vi "BlobSearch.vi"(1 "BlobData R":T2(array[cluster]), 2 "BlobData L":T2(array[cluster])) -> (0 "BlobData":T1(array[cluster]))   [LabVIEW 2011]
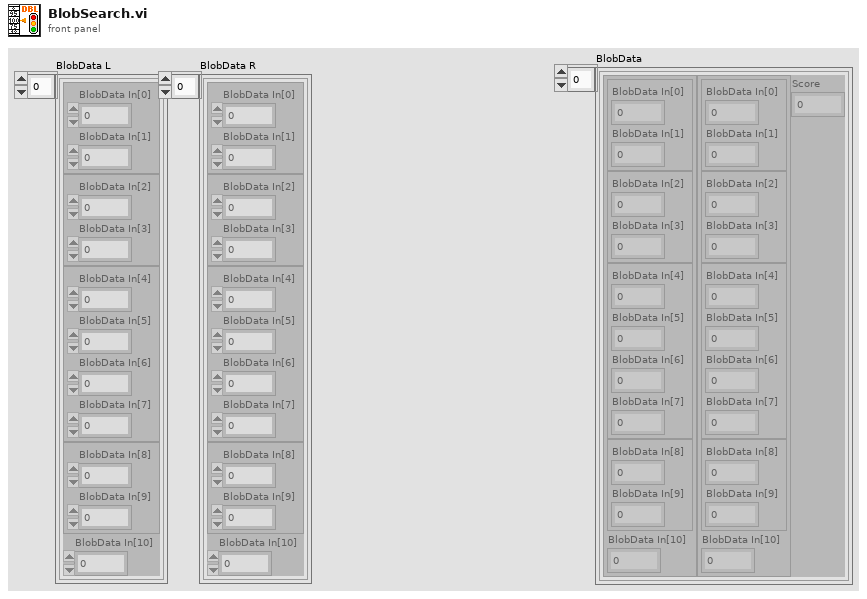
[diagram p1: front panel]
types:
  T1 = cluster{cluster{cluster{"BlobData In[0]":dbl, "BlobData In[1]":dbl}, cluster{"BlobData In[2]":dbl, "BlobData In[3]":dbl}, cluster{"BlobData In[4]":dbl, "BlobData In[5]":dbl, "BlobData In[6]":dbl, "BlobData In[7]":dbl}, cluster{"BlobData In[8]":dbl, "BlobData In[9]":dbl}, "BlobData In[10]":dbl}, cluster{cluster{"BlobData In[0]":dbl, "BlobData In[1]":dbl}, cluster{"BlobData In[2]":dbl, "BlobData In[3]":dbl}, cluster{"BlobData In[4]":dbl, "BlobData In[5]":dbl, "BlobData In[6]":dbl, "BlobData In[7]":dbl}, cluster{"BlobData In[8]":dbl, "BlobData In[9]":dbl}, "BlobData In[10]":dbl}, "Score":dbl}[]
  T2 = cluster{cluster{"BlobData In[0]":dbl, "BlobData In[1]":dbl}, cluster{"BlobData In[2]":dbl, "BlobData In[3]":dbl}, cluster{"BlobData In[4]":dbl, "BlobData In[5]":dbl, "BlobData In[6]":dbl, "BlobData In[7]":dbl}, cluster{"BlobData In[8]":dbl, "BlobData In[9]":dbl}, "BlobData In[10]":dbl}[]
  T3 = cluster{cluster{cluster{"BlobData In[0]":dbl, "BlobData In[1]":dbl}, cluster{"BlobData In[2]":dbl, "BlobData In[3]":dbl}, cluster{"BlobData In[4]":dbl, "BlobData In[5]":dbl, "BlobData In[6]":dbl, "BlobData In[7]":dbl}, cluster{"BlobData In[8]":dbl, "BlobData In[9]":dbl}, "BlobData In[10]":dbl}, cluster{cluster{"BlobData In[0]":dbl, "BlobData In[1]":dbl}, cluster{"BlobData In[2]":dbl, "BlobData In[3]":dbl}, cluster{"BlobData In[4]":dbl, "BlobData In[5]":dbl, "BlobData In[6]":dbl, "BlobData In[7]":dbl}, cluster{"BlobData In[8]":dbl, "BlobData In[9]":dbl}, "BlobData In[10]":dbl}, dbl}[]
  T4 = cluster{cluster{"BlobData In[0]":dbl, "BlobData In[1]":dbl}, cluster{"BlobData In[2]":dbl, "BlobData In[3]":dbl}, cluster{"BlobData In[4]":dbl, "BlobData In[5]":dbl, "BlobData In[6]":dbl, "BlobData In[7]":dbl}, cluster{"BlobData In[8]":dbl, "BlobData In[9]":dbl}, "BlobData In[10]":dbl}
  T5 = cluster{"BlobData In[0]":dbl, "BlobData In[1]":dbl}
  T6 = cluster{"BlobData In[2]":dbl, "BlobData In[3]":dbl}
  T7 = cluster{"BlobData In[4]":dbl, "BlobData In[5]":dbl, "BlobData In[6]":dbl, "BlobData In[7]":dbl}
  T8 = cluster{"BlobData In[8]":dbl, "BlobData In[9]":dbl}
  T9 = cluster{cluster{cluster{"BlobData In[0]":dbl, "BlobData In[1]":dbl}, cluster{"BlobData In[2]":dbl, "BlobData In[3]":dbl}, cluster{"BlobData In[4]":dbl, "BlobData In[5]":dbl, "BlobData In[6]":dbl, "BlobData In[7]":dbl}, cluster{"BlobData In[8]":dbl, "BlobData In[9]":dbl}, "BlobData In[10]":dbl}, cluster{cluster{"BlobData In[0]":dbl, "BlobData In[1]":dbl}, cluster{"BlobData In[2]":dbl, "BlobData In[3]":dbl}, cluster{"BlobData In[4]":dbl, "BlobData In[5]":dbl, "BlobData In[6]":dbl, "BlobData In[7]":dbl}, cluster{"BlobData In[8]":dbl, "BlobData In[9]":dbl}, "BlobData In[10]":dbl}, dbl}
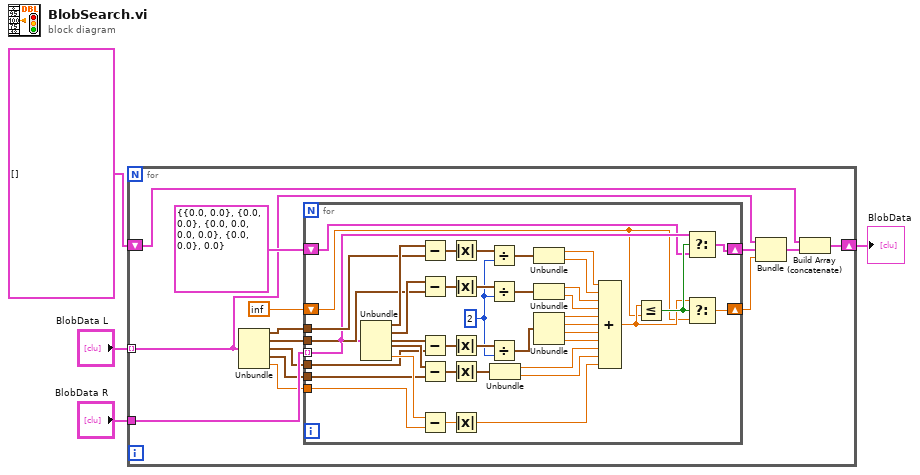
[diagram p0: block diagram]
diagram:
  n1 = for {
    tunnel: "BlobData L" -> [w14] mode=indexing
    tunnel: "BlobData R" -> [w18]
    shift-right: [w11] -> w2
    shift-left: T3 [] -> [w10]
    n2 = Unbundle(w14) -> (w9:T5, w8:T6, w7:T7, w17:T8, "BlobData In[10]"=w16:dbl)
    n3 = for {
      tunnel: w18 -> [w28] mode=indexing
      tunnel: w16 -> [w57]
      tunnel: w17 -> [w55]
      shift-right: [w23] -> w13
      shift-left: T4 {{"BlobData In[0]"=0.0, "BlobData In[1]"=0.0}, {"BlobData In[2]"=0.0, "BlobData In[3]"=0.0}, {"BlobData In[4]"=0.0, "BlobData In[5]"=0.0, "BlobData In[6]"=0.0, "BlobData In[7]"=0.0}, {"BlobData In[8]"=0.0, "BlobData In[9]"=0.0}, "BlobData In[10]"=0.0} -> [w27]
      tunnel: w9 -> [w50]
      tunnel: w8 -> [w49]
      tunnel: w7 -> [w48]
      shift-right: [w24] -> w5
      shift-left: inf -> [w25]
      w19 = 2
      n4 = Unbundle(w28) -> (w53:T5, w52:T6, w51:T7, w59:T8, "BlobData In[10]"=w58:dbl)
      n5 = Subtract(x=w53, y=w50) -> (x-y=w47:T5)
      n6 = Subtract(x=w52, y=w49) -> (x-y=w46:T6)
      n7 = Subtract(x=w51, y=w48) -> (x-y=w45:T7)
      n8 = Subtract(x=w59, y=w55) -> (x-y=w56:T8)
      n9 = Subtract(x=w58, y=w57) -> (x-y=w54:dbl)
      n10 = Absolute Value(x=w47) -> (abs(x)=w44:T5)
      n11 = Absolute Value(x=w46) -> (abs(x)=w43:T6)
      n12 = Absolute Value(x=w45) -> (abs(x)=w42:T7)
      n13 = Absolute Value(x=w56) -> (abs(x)=w33:T8)
      n14 = Absolute Value(x=w54) -> (abs(x)=w30:dbl)
      n15 = Divide(x=w44, y=w19) -> (x/y=w22:T5)
      n16 = Divide(x=w43, y=w19) -> (x/y=w21:T6)
      n17 = Divide(x=w42, y=w19) -> (x/y=w20:T7)
      n18 = Unbundle(w33) -> ("BlobData In[8]"=w32:dbl, "BlobData In[9]"=w31:dbl)
      n19 = Unbundle(w22) -> ("BlobData In[0]"=w41:dbl, "BlobData In[1]"=w40:dbl)
      n20 = Unbundle(w21) -> ("BlobData In[2]"=w39:dbl, "BlobData In[3]"=w38:dbl)
      n21 = Unbundle(w20) -> ("BlobData In[4]"=w37:dbl, "BlobData In[5]"=w36:dbl, "BlobData In[6]"=w35:dbl, "BlobData In[7]"=w34:dbl)
      n22 = Compound Arithmetic op=ADD(w41, w40, w39, w38, w37, w36, w35, w34, w32, w31, w30) -> (w26:dbl)
      n23 = Less Or Equal?(x=w26, y=w25) -> (x <= y?=w29:bool)
      n24 = Select(t=w28, s=w29, f=w27) -> (s? t:f=w23:T4)
      n25 = Select(t=w26, s=w29, f=w25) -> (s? t:f=w24:dbl)
    }
    n26 = Bundle(w14, w13, w5) -> (w12:T9)  [unwired: 1 in]
    n27 = Build Array (concatenate)(w10, w12) -> (w11:T3)
  }
  "BlobData" <- w2
